vi "Update All Values.vi"(8 "error in (no error)":errorcluster, 10 "Values":refnum<class "Type.lvclass">[](array[class]), 11 "NewEntityTemplate in":refnum<class "NewEntityTemplate.lvclass">) -> (0 "error out":errorcluster, 3 "NewEntityTemplate out":refnum<class "NewEntityTemplate.lvclass">)   [LabVIEW 2020, in "Conditum-Tools.lvlib" / "NewEntityTemplate.lvclass"]
uses:
  NewEntityTemplate.lvclass
  Conditum/Columns/Type/Type.lvclass
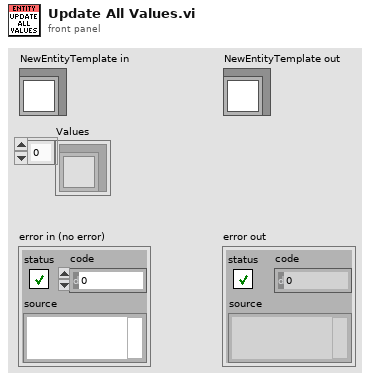
[diagram p1: front panel]
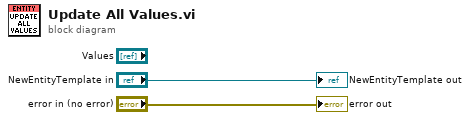
[diagram p0: block diagram]
diagram:
  "error out" <- "error in (no error)"
  "NewEntityTemplate out" <- "NewEntityTemplate in"
